vi "Close VI.vi"(10 "VI Refnum":refnum<vi>, 11 "App Ref":refnum<vi>) -> ()   [LabVIEW 2024, in "Wordle Scorer.lvlib"]
uses:
  Wordle Scorer.lvlib
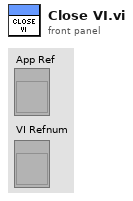
[diagram p1: front panel]
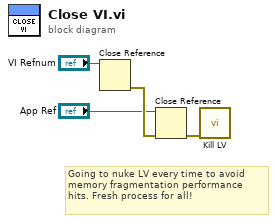
[diagram p0: block diagram]
diagram:
  # "Going to nuke LV every time to avoid memory fragmentation performance hits. Fresh process for all!"
  n1 = Close Reference(reference="VI Refnum") -> (error out=w4:errorcluster)  [unwired: 1 in]
  n2 = Close Reference(reference="App Ref", error in (no error)=w4) -> (error out=w1:errorcluster)
  n3 = call "Kill LV.vi"("error in (no error)"=w1) -> ()  [unwired: 9 in, 2 out]
